vi "Library Initialize and Exit.vi"(7 "action":enum16{"LibInit", "LibExit"}(ring), 8 "error in":errorcluster) -> (0 "error out":errorcluster, 3 "instance count":u32)   [LabVIEW 2020, in "AIM MIL-STD-1553 Hardware API.lvlib"]
uses:
  AIM MIL-STD-1553 Hardware API.lvlib
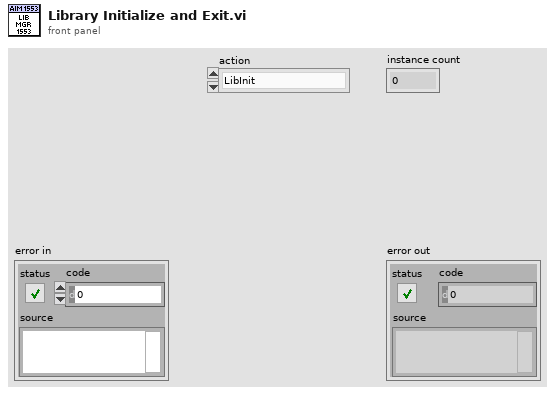
[diagram p1: front panel]
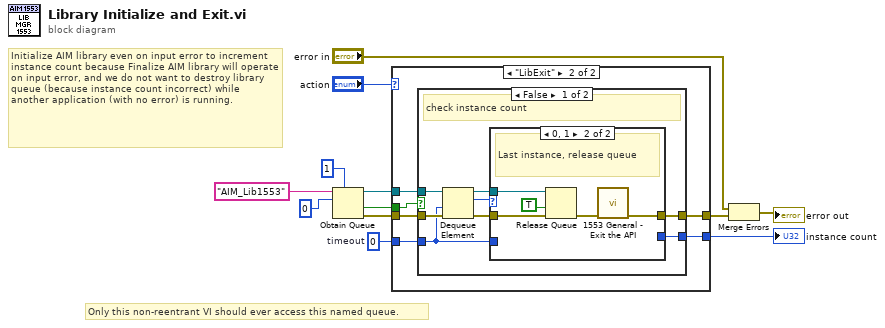
[diagram p0: block diagram]
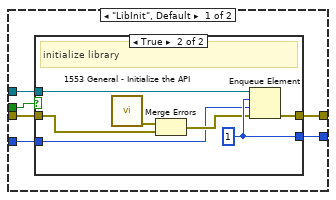
[diagram p2: hidden frame]
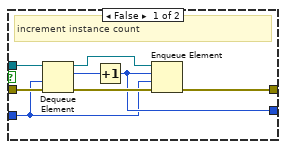
[diagram p3: hidden frame]
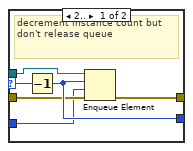
[diagram p4: hidden frame]
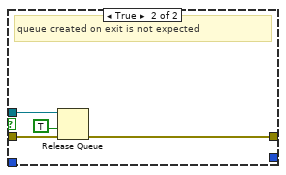
[diagram p5: hidden frame]
diagram:
  w1 = 0  # timeout
  # "Initialize AIM library even on input error to increment instance count because Finalize AIM library will operate on input error, and we do not want to destroy library queue (because instance count incorrect) while another application (with no error) is running."
  # "Only this non-reentrant VI should ever access this named queue."
  n1 = Obtain Queue(max queue size (-1, unlimited)=1, name (unnamed)="AIM_Lib1553", element data type=u32 0) -> (queue out=w4:refnum<queue>, created new?=w3:bool, error out=w2:errorcluster)  [unwired: 2 in]
  n2 = case shown="\"LibExit\"" "action" {
    tunnel: [w18 w39] -> w11
    tunnel: [w17 w38] -> w12
    tunnel: w4 -> [w16 w37]
    tunnel: w3 -> [w15 w36]
    tunnel: w2 -> [w14 w35]
    tunnel: w1 -> [w13 w34]
    frame "LibInit", Default {
      n3 = case shown="True" w15 {
        tunnel: w14 -> [w25 w29]
        tunnel: [w22 w33] -> w18
        tunnel: [w21 w31] -> w17
        tunnel: w16 -> [w26 w32]
        tunnel: w13 -> [w19 w27]
        frame False {
          # "increment instance count"
          n4 = Dequeue Element(queue=w26, timeout in ms (-1)=w19, error in (no error)=w25) -> (queue out=w24:refnum<queue>, element=w20:u32, error out=w23:errorcluster)  [unwired: 1 out]
          n5 = Increment(x=w20) -> (x+1=w21:u32)
          n6 = Enqueue Element(queue=w24, element=w21, timeout in ms (-1)=w19, error in (no error)=w23) -> (error out=w22:errorcluster)  [unwired: 2 out]
        }
        frame True {
          w31 = u32 1 ("modules found")
          # "initialize library"
          n7 = call <instrlib>:"1553 General - Initialize the API.vi"() -> ("Error Out"=w28:errorcluster)  [unwired: 10 in, 1 out]
          n8 = Merge Errors(w28, w29) -> (w30:errorcluster)
          n9 = Enqueue Element(queue=w32, element=w31, timeout in ms (-1)=w27, error in (no error)=w30) -> (error out=w33:errorcluster)  [unwired: 2 out]
        }
      }
    }
    frame "LibExit" {
      n10 = case shown="False" w36 {
        tunnel: [w47 w60] -> w39
        tunnel: [w46 _] -> w38
        tunnel: w37 -> [w45 w62]
        tunnel: w35 -> [w44 w61]
        tunnel: w34 -> [w40 _]
        frame False {
          # "check instance count"
          n11 = Dequeue Element(queue=w45, timeout in ms (-1)=w40, error in (no error)=w44) -> (queue out=w42:refnum<queue>, element=w43:u32, error out=w41:errorcluster)  [unwired: 1 out]
          n12 = case shown="0, 1" w43 {
            selector: w43 -> [w51 _]
            tunnel: [w52 w55] -> w47
            tunnel: [w53 _] -> w46
            tunnel: w42 -> [w50 w58]
            tunnel: w41 -> [w49 w57]
            tunnel: w40 -> [w48 _]
            frame 2.. {
              # "decrement instance count but don't release queue"
              n13 = Decrement(x=w51) -> (x-1=w53:u32)
              n14 = Enqueue Element(queue=w50, element=w53, timeout in ms (-1)=w48, error in (no error)=w49) -> (error out=w52:errorcluster)  [unwired: 2 out]
            }
            frame 0, 1 {
              # "Last instance, release queue"
              n15 = Release Queue(queue=w58, force destroy? (F)=TRUE, error in (no error)=w57) -> (error out=w56:errorcluster)  [unwired: 2 out]
              n16 = call <instrlib>:"1553 General - Exit the API.vi"("Error In (none)"=w56) -> ("Error Out"=w55:errorcluster)  [unwired: 10 in]
            }
          }
        }
        frame True {
          # "queue created on exit is not expected"
          n17 = Release Queue(queue=w62, force destroy? (F)=TRUE, error in (no error)=w61) -> (error out=w60:errorcluster)  [unwired: 2 out]
        }
      }
    }
  }
  "instance count" <- w12
  n18 = Merge Errors("error in", w11) -> (→"error out":errorcluster)
